vi "Close.vi"(8 "error in (no error)":errorcluster, 11 "reference in":refnum<class "Object_Editor.lvclass">) -> (0 "error out":errorcluster, 3 "reference in":refnum<class "Object_Editor.lvclass">)   [LabVIEW 2022 SP3, in "Object_Editor.lvlib" / "Object_Editor.lvclass"]
uses:
  Object_Editor.lvclass
  Components/ViPER.lvlibp/ViPER.lvclass
  C:/Projects/Medulla/ViPER/ViPER_ProjectTemplates/ProjectTemplates/Source/Core/ViPER/Components/ViPER.lvlibp/ViPER.lvclass
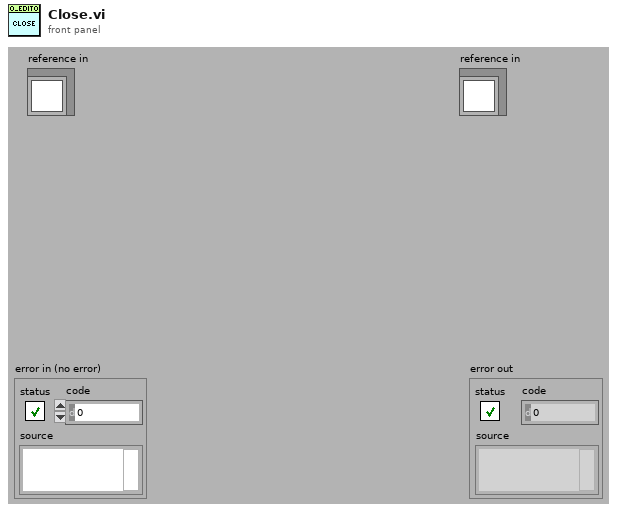
[diagram p1: front panel]
types:
  T1 = typedef "Object_Editor.lvlib/Object_Editor.lvclass/ObjectAttributes.ctl" = cluster{"Config":T2, "Tree":refnum<vi>, "Mod_Bit":bool, "File_Path":path, "Object":refnum<class "ViPER.lvclass">}
  T2 = typedef "Object_Editor.lvlib/Object_Editor.lvclass/Config.ctl" = cluster{"default":string}
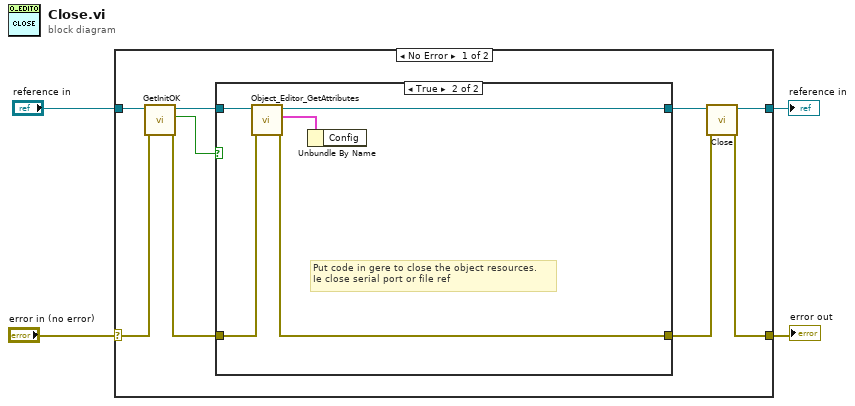
[diagram p0: block diagram]
diagram:
  n1 = case shown="No Error" "error in (no error)" {
    selector: "error in (no error)" -> [w6 w22]
    tunnel: [w11 w22] -> w3
    tunnel: [w12 w21] -> w1
    tunnel: "reference in" -> [w9 w21]
    frame No Error {
      n2 = call "GetInitOK.vi"("error in (no error)"=w6, "reference in"=w9) -> ("error out"=w5:errorcluster, "init_ok"=w7:bool, "reference out"=w8:refnum<class "Object_Editor.lvclass">)  [unwired: 7 in]
      n3 = case shown="True" w7 {
        tunnel: w5 -> [w15 w19]
        tunnel: [w15 w18] -> w10
        tunnel: w8 -> [w14 w20]
        tunnel: [w14 w16] -> w13
        frame False {
        }
        frame True {
          # "Put code in gere to close the object resources.\nIe close serial port or file ref"
          n4 = call "Object_Editor_GetAttributes.vi"("error in (no error)"=w19, "reference in"=w20) -> ("error out"=w18:errorcluster, "Data"=w17:T1, "reference out"=w16:refnum<class "Object_Editor.lvclass">)  [unwired: 6 in, 1 out]
          n5 = Unbundle By Name(w17) -> ()  [unwired: 1 out]
        }
      }
      n6 = call-parent "Close.vi"("error in (no error)"=w10, "reference in"=w13) -> ("error out"=w11:errorcluster, "reference out"=w12:refnum<class "Object_Editor.lvclass">)  [unwired: 8 in]
    }
    frame Error {
    }
  }
  "error out" <- w3
  "reference in" <- w1
